vi "FTW-ProjectItemManager-RegisterMailbox.vi"(0 "Project Item Manager":refnum<class "FTW-ProjectItemManager.lvclass">, 11 "error in":errorcluster) -> (4 "Project Item Manager out":refnum<class "FTW-ProjectItemManager.lvclass">, 6 "Property Change Event":refnum<event-registration>, 15 "error out":errorcluster)   [LabVIEW 2012, in "FTW-ProjectItemManager.lvclass"]
uses:
  FTW-ProjectItemManager.lvclass
  Core/Messaging/Message/FTW-Message.lvclass
  FTW-ProjectItemManager.lvclass/FTW-ProjectItemManager.ctl
  Core/Messaging/Messenger/FTW-Messenger.lvclass
panel:
  # "Inputs"
  # "Outputs"
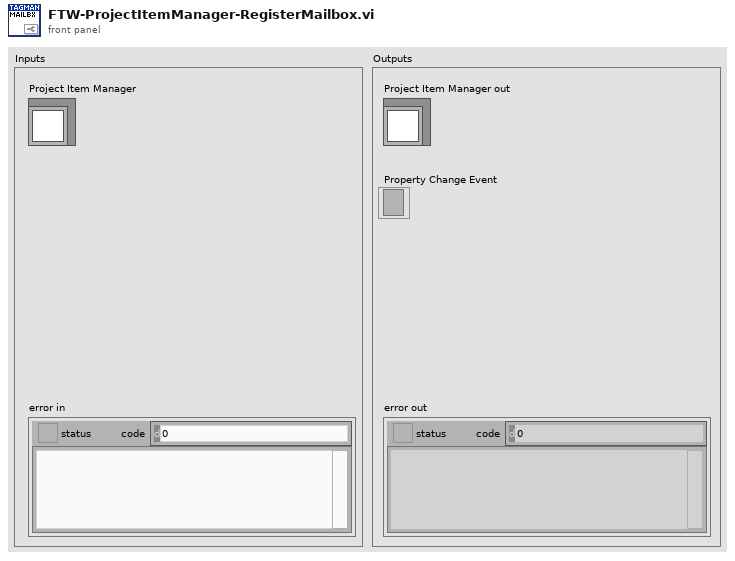
[diagram p1: front panel]
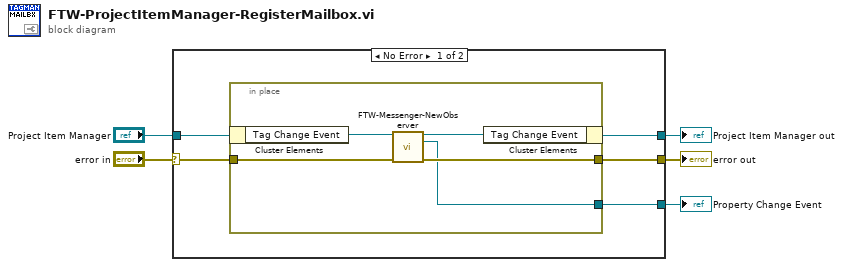
[diagram p0: block diagram]
diagram:
  n1 = case shown="No Error" "error in" {
    selector: "error in" -> [w8 w17]
    tunnel: [w10 w17] -> w5
    tunnel: [w6 w16] -> w3
    tunnel: "Project Item Manager" -> [w7 w16]
    tunnel: [w9 _] -> w1
    frame No Error {
      n2 = in-place {
        in-place-border: [w15] -> w10
        in-place-border: [w14] -> w9
        in-place-border: w8 -> [w13]
        n3 = in-place-cluster #1(w7) -> ("Tag Change Event"=w12:refnum<class "FTW-Messenger-Actor.lvclass">)
        n4 = call "FTW-Messenger-NewObserver.vi"("Messenger"=w12, "error in"=w13) -> ("Messenger out"=w11:refnum<class "FTW-Messenger-Actor.lvclass">, "Message"=w14:refnum<event-registration>, "error out"=w15:errorcluster)  [unwired: 11 in]
        n5 = in-place-cluster #1("Tag Change Event"=w11) -> (w6:refnum<class "FTW-ProjectItemManager.lvclass">)
      }
    }
    frame Error {
    }
  }
  "error out" <- w5
  "Project Item Manager out" <- w3
  "Property Change Event" <- w1
